vi "Monedas.vi"(8 "error in (no error)":errorcluster, 10 "Monedas":T1, 11 "Actor_C_MXN in":refnum<class "Actor_C_MXN.lvclass">) -> (0 "error out":errorcluster, 3 "Actor_C_MXN out":refnum<class "Actor_C_MXN.lvclass">)   [LabVIEW 2019, in "Actor_C_MXN.lvlib" / "Actor_C_MXN.lvclass"]
uses:
  Actor_C_MXN.lvclass
  C:/Program Files/National Instruments/LabVIEW 2019/vi.lib/ActorFramework/Actor/Actor.lvclass
  <vilib>/ActorFramework/Actor/Actor.lvclass/Actor.ctl
  Actor_C_MXN.lvclass/Actor_C_MXN.ctl
  UI Actor Messages/Update Credit Msg/Update Credit Msg.lvclass/Update Credit Msg.ctl
  <vilib>/ActorFramework/Message Enqueuer/Message Enqueuer.lvclass/Message Enqueuer.ctl
  <vilib>/ActorFramework/Message Enqueuer/Enqueue.vi
  UI Actor Messages/Update Credit Msg/Update Credit Msg.lvclass
  C:/Program Files/National Instruments/LabVIEW 2019/vi.lib/ActorFramework/Message/Message.lvclass
  <vilib>/ActorFramework/Message Priority Queue/Priority Enqueue.vi
  <vilib>/ActorFramework/Actor/Actor.lvclass
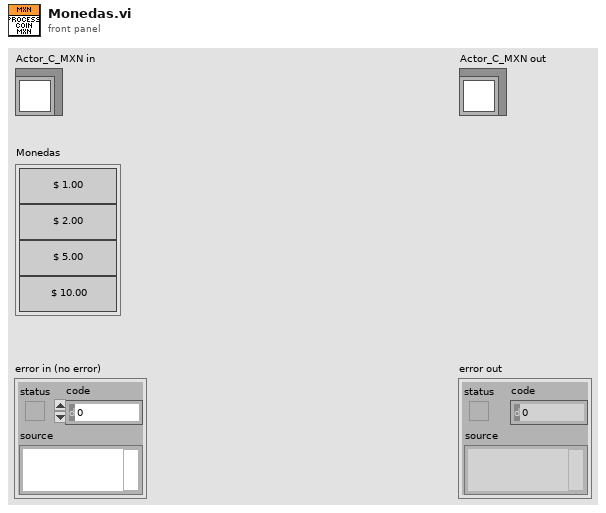
[diagram p1: front panel]
types:
  T1 = cluster{"1 P":bool, "2 P":bool, "5P":bool, "10 P":bool}
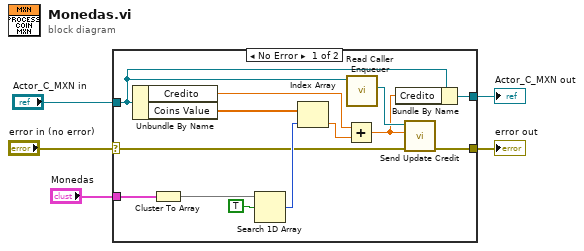
[diagram p0: block diagram]
diagram:
  n1 = case shown="No Error" "error in (no error)" {
    selector: "error in (no error)" -> [w7 w20]
    tunnel: [w6 w20] -> w4
    tunnel: [w11 w19] -> w2
    tunnel: "Actor_C_MXN in" -> [w10 w19]
    tunnel: "Monedas" -> [w18 _]
    frame No Error {
      n2 = Unbundle By Name(w10) -> ("Credito"=w13:dbl, "Coins Value"=w14:dbl[])
      n3 = Cluster To Array(cluster=w18) -> (array=w17:bool[])
      n4 = Search 1D Array(1D array=w17, element=TRUE) -> (index of element=w15:i32)  [unwired: 1 in]
      n5 = Index Array(array=w14, index=w15) -> (element=w12:dbl)
      n6 = Add(x=w13, y=w12) -> (x+y=w8:dbl)
      n7 = call <vilib>:"Read Caller Enqueuer.vi"("Actor"=w10) -> ("Caller Enqueuer"=w9:refnum<class "Message Enqueuer.lvclass">)  [unwired: 10 in]
      n8 = Bundle By Name(cluster=w10, "Credito"=w8) -> (w11:refnum<class "Actor_C_MXN.lvclass">)
      n9 = call "Send Update Credit.vi"("error in (no error)"=w7, "Credito"=w8, "Message Enqueuer"=w9) -> ("error out"=w6:errorcluster)  [unwired: 7 in, 1 out]
    }
    frame Error {
    }
  }
  "error out" <- w4
  "Actor_C_MXN out" <- w2
